vi "Handle Error.vi"(8 "error in (no error)":errorcluster, 11 "WebSocket Client in":refnum<class "WebSocket Client.lvclass">) -> (0 "error out":errorcluster, 2 "stop actor?":bool=TRUE, 3 "WebSocket Client out":refnum<class "WebSocket Client.lvclass">)   [LabVIEW 2021, in "WebSocket Actors.lvlib" / "WebSocket Client.lvclass"]
doc: "(<B>Filename</B>: Actor Framework.lvlib:Actor.lvclass:Handle Error.vi)\n\nDefines how the actor handles an error that occurred while processing a message. By default, this method does nothing except stop the actor."
uses:
  WebSocket Client.lvclass
  WebSocket Client.lvclass/WebSocket Client.ctl
  <vilib>/ActorFramework/Report Error Msg/Report Error Msg.lvclass
  <userlib>/_OpenG.lib/error/error.llb/openg_error.lvlib
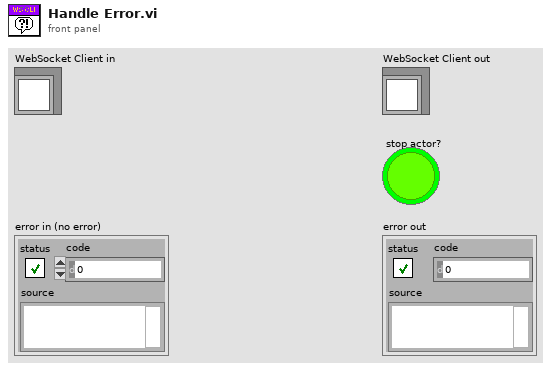
[diagram p1: front panel]
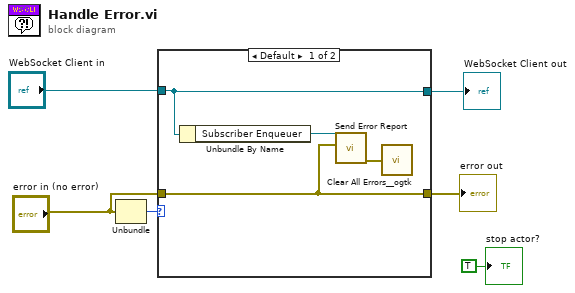
[diagram p0: block diagram]
diagram:
  n1 = Unbundle("error in (no error)") -> ("code"=w6:i32)  [unwired: 2 out]
  n2 = case shown="Default" w6 {
    tunnel: [w9 _] -> w4
    tunnel: "error in (no error)" -> [w9 _]
    tunnel: "WebSocket Client in" -> [w7 w11]
    tunnel: [w7 w11] -> w1
    frame Default {
      n3 = Unbundle By Name(w7) -> ("Subscriber Enqueuer"=w10:refnum<class "Message Enqueuer.lvclass">)
      n4 = call <vilib>:"Send Error Report.vi"("Error From Sender"=w9, "Message Enqueuer"=w10) -> ("error out"=w8:errorcluster)  [unwired: 9 in]
      n5 = call <userlib>:"Clear All Errors__ogtk.vi"("Error In"=w8) -> ()  [unwired: 3 in, 1 out]
    }
    frame 43 {
      # "\"Cancel Error\" means stop, but \"No Error\" to caller."
    }
  }
  "WebSocket Client out" <- w1
  "error out" <- w4
  "stop actor?" <- TRUE ("stop actor?")
